vi "szeregowe i rownolegle.vi"() -> ()   [LabVIEW 2013]
panel:
  out "opoznienie 2":dbl
  in  "stop 2":bool
  in  "stop":bool
  out "opoznienie":dbl
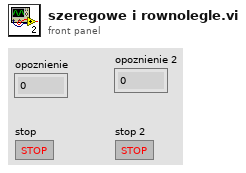
[diagram p1: front panel]
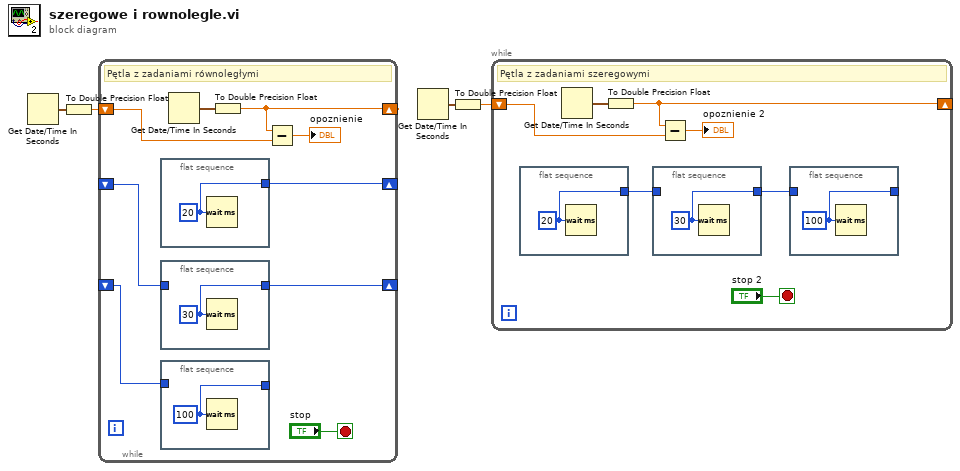
[diagram p0: block diagram]
diagram:
  n1 = Get Date/Time In Seconds() -> (seconds since 1Jan1904=w4:timestamp)
  n2 = To Double Precision Float(number=w4) -> (double precision float=w3:dbl)
  n3 = while {
    shift-right: [w12] -> _
    shift-left: w3 -> [w11]
    shift-right: [w5] -> _
    shift-left: _ -> [w8]
    shift-right: [w7] -> _
    shift-left: _ -> [w6]
    stop <- "stop" stop-if-true
    # "Pętla z zadaniami równoległymi"
    n4 = flat-sequence {
      tunnel: [w16] -> w5
      frame #0 {
        w16 = u32 20 ("milliseconds to wait")
        n5 = Wait (ms)(milliseconds to wait=w16) -> ()  [unwired: 1 out]
      }
    }
    n6 = flat-sequence {
      tunnel: [w15] -> w7
      tunnel: w8 -> [_]
      frame #0 {
        w15 = u32 30 ("milliseconds to wait")
        n7 = Wait (ms)(milliseconds to wait=w15) -> ()  [unwired: 1 out]
      }
    }
    n8 = flat-sequence {
      tunnel: [w14] -> _
      tunnel: w6 -> [_]
      frame #0 {
        w14 = u32 100 ("milliseconds to wait")
        n9 = Wait (ms)(milliseconds to wait=w14) -> ()  [unwired: 1 out]
      }
    }
    n10 = Get Date/Time In Seconds() -> (seconds since 1Jan1904=w13:timestamp)
    n11 = To Double Precision Float(number=w13) -> (double precision float=w12:dbl)
    n12 = Subtract(x=w12, y=w11) -> (x-y=→"opoznienie":dbl)
  }
  n13 = Get Date/Time In Seconds() -> (seconds since 1Jan1904=w1:timestamp)
  n14 = To Double Precision Float(number=w1) -> (double precision float=w2:dbl)
  n15 = while {
    shift-right: [w22] -> _
    shift-left: w2 -> [w21]
    stop <- "stop 2" stop-if-true
    # "Pętla z zadaniami szeregowymi"
    n16 = flat-sequence {
      tunnel: [w26] -> w18
      frame #0 {
        w26 = u32 20 ("milliseconds to wait")
        n17 = Wait (ms)(milliseconds to wait=w26) -> ()  [unwired: 1 out]
      }
    }
    n18 = Get Date/Time In Seconds() -> (seconds since 1Jan1904=w23:timestamp)
    n19 = To Double Precision Float(number=w23) -> (double precision float=w22:dbl)
    n20 = flat-sequence {
      tunnel: [w25] -> w17
      tunnel: w18 -> [_]
      frame #0 {
        w25 = u32 30 ("milliseconds to wait")
        n21 = Wait (ms)(milliseconds to wait=w25) -> ()  [unwired: 1 out]
      }
    }
    n22 = Subtract(x=w22, y=w21) -> (x-y=→"opoznienie 2":dbl)
    n23 = flat-sequence {
      tunnel: [w24] -> _
      tunnel: w17 -> [_]
      frame #0 {
        w24 = u32 100 ("milliseconds to wait")
        n24 = Wait (ms)(milliseconds to wait=w24) -> ()  [unwired: 1 out]
      }
    }
  }
